vi "20170502-lecture4-1 write to file binary.vi"() -> ()   [LabVIEW 2014]
panel:
  out "number (0 to 1)":dbl
  in  "Path":path
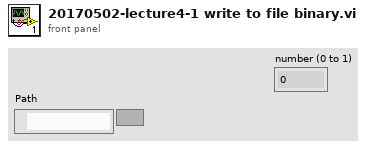
[diagram p1: front panel]
types:
  T1 = enum16{"open", "replace", "create", "open or create", "replace or create", "replace or create with confirmation"}
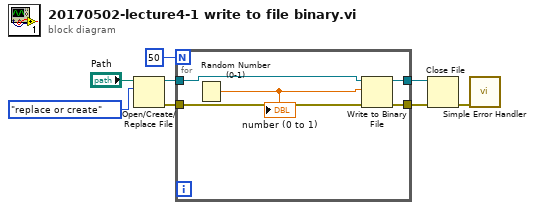
[diagram p0: block diagram]
diagram:
  n1 = Open/Create/Replace File(file path (use dialog)="Path", operation (0:open)=T1."replace or create") -> (refnum out=w7:refnum<file>, error out=w2:errorcluster)  [unwired: 4 in, 1 out]
  n2 = for {
    N: 50 -> [_]
    tunnel: w7 -> [w12]
    tunnel: [w11] -> w5
    tunnel: [w10] -> w3
    tunnel: w2 -> [w9]
    n3 = Random Number (0-1)() -> (number: 0 to 1=w13:dbl)
    "number (0 to 1)" <- w13
    n4 = Write to Binary File(file (use dialog)=w12, data=w13, error in=w9) -> (refnum out=w11:refnum<file>, error out=w10:errorcluster)  [unwired: 3 in, 1 out]
  }
  n5 = Close File(refnum=w5, error in=w3) -> (error out=w4:errorcluster)  [unwired: 1 out]
  n6 = call <vilib>:"Simple Error Handler.vi"("error in (no error)"=w4) -> ()  [unwired: 4 in, 5 out]
